vi "PPAS-simulate-dashboard.vi"() -> ()   [LabVIEW 2019]
uses:
  Swerve_Drive_System/PPAS_DRIVE_GLOBALS.vi
  Simulation/PPAS_SIM_SIM_Globals.vi
  AutoCommand/PPAS_AUTOCMD_GLOBALS.vi
  <vilib>/Rock Robotics/WPI/ThirdParty/JAS_Junk/TrajLib/Trajectory_Library.lvlib
  Vision_Interface/PPAS_Vision_Globals.vi
  CommandProcessing/PPAS_Command_Globals.vi
  <vilib>/Rock Robotics/WPI/ThirdParty/JAS_Junk/TrajLib/TypeDef/ROTATION2D.ctl
  <vilib>/Rock Robotics/WPI/ThirdParty/JAS_Junk/TrajLib/TypeDef/CHASSIS_SPEEDS.ctl
  <vilib>/Rock Robotics/WPI/ThirdParty/JAS_Junk/TrajLib/TypeDef/TRANSLATION2D.ctl
  <vilib>/Rock Robotics/WPI/ThirdParty/JAS_Junk/TrajLib/TypeDef/POSE2D.ctl
panel:
  in  "Tab Control":T1(tab)
  out "Mod Swerve in Deadband 2":bool
  out "Battery Voltage":dbl(graph)
  out "Swerve Motor Demands":T2(graph)
  out "Drive Motor Demands":T2(graph)
  out "Swerve Module Devices":T3(array[cluster])
  out "GyroReading_Degreees":dbl format="%15.3f"
  out "Encoder Distances":dbl[](array[numeric]) format="%17.2f"
  out "Encoder Velocities":dbl[](array[numeric]) format="%17.2f"
  out "Motor Demands":dbl[](array[numeric]) format="%17.2f"
  out "Battery Volts":dbl format="%16.2f"
  out "Mod Wheel \nSpeed Dmd":dbl[](array[numeric]) format="%17.3f"
  out "Swerve Drive Motor output":T4(graph)
  out "Swerve Drive Speed M/S":T5(graph)
  out "Swerve Drive Speed Error  M/S":T6(graph)
  out "Closed Loop Control":bool
  out "Orientation Angle Dmd_Rad":dbl format="%17.3f"
  out "Drv Chassis Adj Velocity DmD":T7 {"vOmega" format="%10.3f"; "vY" format="%10.3f"; "vX" format="%10.3f"}
  out "GyroHeading_Radians":dbl format="%17.2f"
  out "Orientation Angle Error_Rad":dbl format="%17.3f"
  out "Orientation Correct CO":dbl format="%17.3f"
  out "Swerve Chassis Speed":T7 {"vOmega" format="%10.3f"; "vY" format="%10.3f"; "vX" format="%10.3f"}
  out "Mod Swerve in Deadband":bool
  out "Mod Wheel Out":dbl[](array[numeric]) format="%17.3f"
  out "Mod Wheel \nSpeed M/S":dbl[](array[numeric]) format="%17.3f"
  out "Mod Wheel Speed Err":dbl[](array[numeric]) format="%17.3f"
  out "Opt Mod Wheel \nSpeed Dmd":dbl[](array[numeric]) format="%17.3f"
  out "Swerve Pos Dmd\nRadians":dbl[](array[numeric]) format="%17.3f"
  out "Optimized Swerve\nPos Dmd":dbl[](array[numeric]) format="%17.3f"
  out "Sweve Module Motor Output":T8(graph)
  out "Swerve Modue Position Radians":T5(graph)
  out "Swerve Module Position Error\nRadians":T9(graph)
  out "Closed Loop Control 2":bool
  out "Mod Swerve in Deadband 3":bool
  out "Mod Swerve Err  Radians":dbl[](array[numeric]) format="%17.3f"
  out "Mod Swerve Motor Out":dbl[](array[numeric]) format="%17.3f"
  out "Mod Pos Radians":dbl[](array[numeric]) format="%17.3f"
  out "Mod Swerve On Targ":bool[](array[boolean])
  out "Cmd 3":bool
  out "Cmd 2":bool
  out "Cmd 1":bool
  out "Vision Pose":T10={"TRANSLATION"={"X"=0.0, "Y"=0.0}, "ROTATION"={"VALUE"=0.0, "COS"=1.0, "SIN"=0.0}} {"ROTATION"."SIN" format="%13.4f"; "ROTATION"."COS" format="%13.4f"; "ROTATION"."VALUE" format="%13.4f"; "TRANSLATION"."Y" format="%14.3f"; "TRANSLATION"."X" format="%14.3f"}
  out "Vision\nPose":bool
  out "Trajectory Status":T13(graph)
  out "Trajectory Execution \nClosed Loop":bool
  out "Mod Swerve in \nDeadband 3":bool
  out "Trajectory Error":T14(graph)
  out "Traj_OnTarget":bool
  out "Traj Heading Dmd Deg":dbl format="%17.2f"
  out "Traj Final Heading Dmd Deg":dbl format="%17.2f"
  out "Traj Sample Time Sec":dbl format="%17.2f"
  out "Traj Rot Vel FF Rad/Sec":dbl format="%17.2f"
  out "Absolute Odometry \nPose":T10={"TRANSLATION"={"X"=0.0, "Y"=0.0}, "ROTATION"={"VALUE"=0.0, "COS"=1.0, "SIN"=0.0}} {"ROTATION"."SIN" format="%13.4f"; "ROTATION"."COS" format="%13.4f"; "ROTATION"."VALUE" format="%13.4f"; "TRANSLATION"."Y" format="%14.3f"; "TRANSLATION"."X" format="%14.3f"}
  out "Other ABS Odometry\nPose":T10={"TRANSLATION"={"X"=0.0, "Y"=0.0}, "ROTATION"={"VALUE"=0.0, "COS"=1.0, "SIN"=0.0}} {"ROTATION"."SIN" format="%13.4f"; "ROTATION"."COS" format="%13.4f"; "ROTATION"."VALUE" format="%13.4f"; "TRANSLATION"."Y" format="%14.3f"; "TRANSLATION"."X" format="%14.3f"}
  # "SIMULATION"
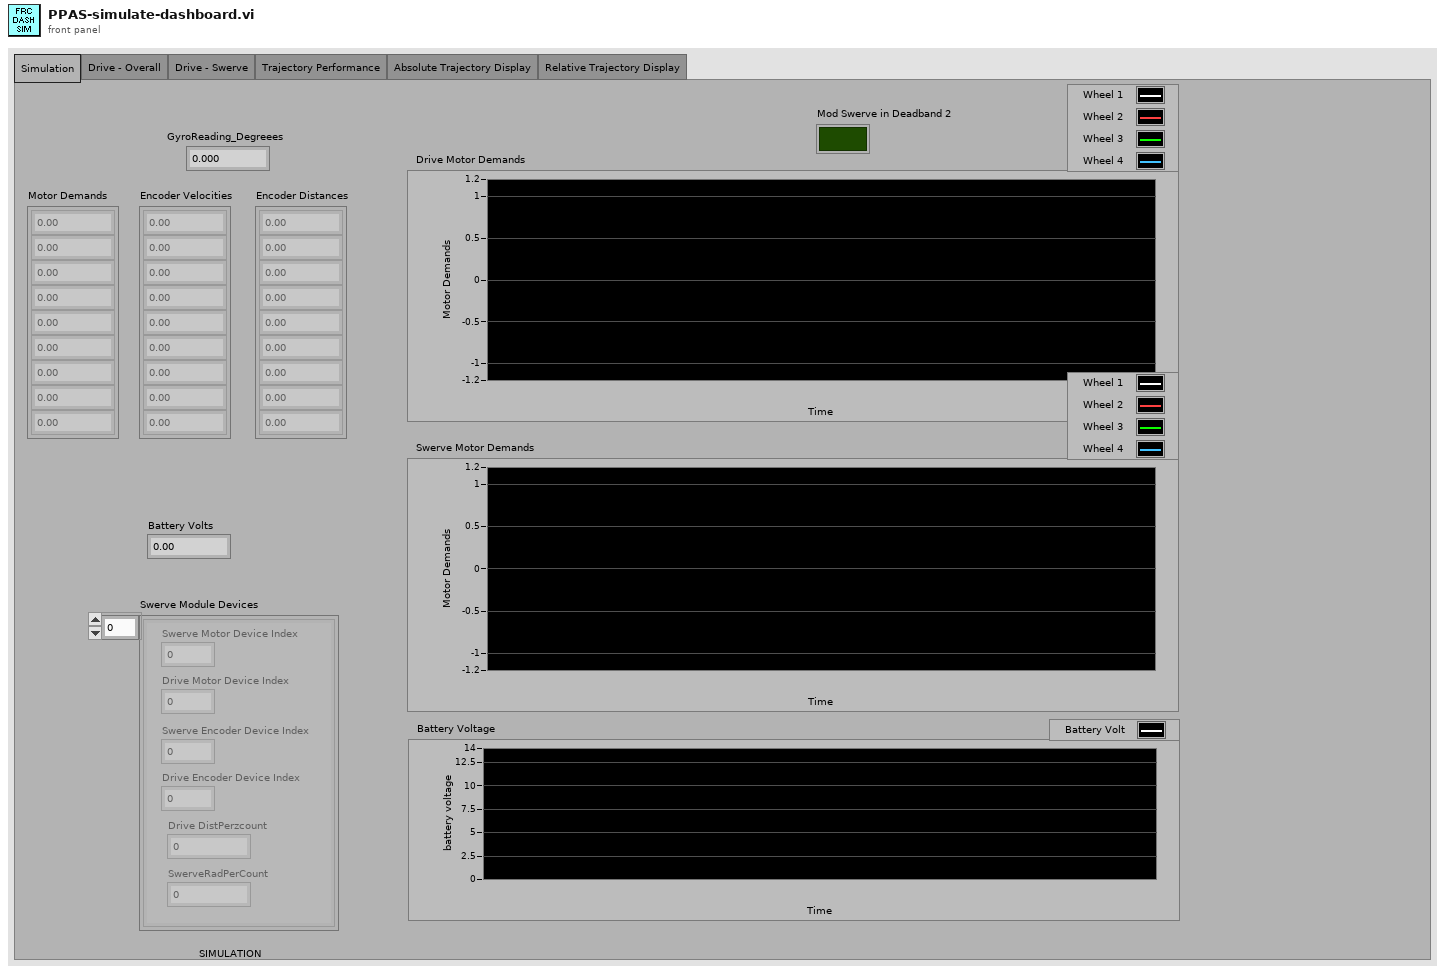
[diagram p1: front panel]
types:
  T1 = enum32{"Simulation", "Drive - Overall", "Drive - Swerve", "Trajectory Performance", "Absolute Trajectory Display", "Relative Trajectory Display"}
  T2 = cluster{"Motor Dmd":dbl, "Motor Dmd":dbl, "Motor Dmd":dbl, "Motor Dmd":dbl}
  T3 = cluster{"Swerve Motor Device Index":i32, "Drive Motor Device Index":i32, "Swerve Encoder Device Index":i32, "Drive Encoder Device Index":i32, "Drive DistPerzcount":dbl, "SwerveRadPerCount":dbl}[]
  T4 = cluster{"Mod Wheel Out[0]":dbl, "Mod Wheel Out[1]":dbl, "Mod Wheel Out[2]":dbl, "Mod Wheel Out[3]":dbl}
  T5 = cluster{"Angle RADIANS":dbl, "Angle RADIANS":dbl, "Angle RADIANS":dbl, "Distance M":dbl}
  T6 = cluster{"Mod Wheel Speed Err[0]":dbl, "Mod Wheel Speed Err[1]":dbl, "Mod Wheel Speed Err[2]":dbl, "Mod Wheel Speed Err[3]":dbl}
  T7 = typedef "Trajectory_Library.lvlib/CHASSIS_SPEEDS.ctl" = cluster{"vX":dbl, "vY":dbl, "vOmega":dbl}
  T8 = cluster{"Mod Swerve Out[0]":dbl, "Mod Swerve Out[1]":dbl, "Mod Swerve Out[2]":dbl, "Mod Swerve Out[3]":dbl}
  T9 = cluster{"Mod Swerve Err[0]":dbl, "Mod Swerve Err[1]":dbl, "Mod Swerve Err[2]":dbl, "Mod Swerve Err[3]":dbl}
  T10 = typedef "Trajectory_Library.lvlib/POSE2D.ctl" = cluster{"TRANSLATION":T11, "ROTATION":T12}
  T11 = typedef "Trajectory_Library.lvlib/TRANSLATION2D.ctl" = cluster{"X":dbl, "Y":dbl}
  T12 = typedef "Trajectory_Library.lvlib/ROTATION2D.ctl" = cluster{"VALUE":dbl, "COS":dbl, "SIN":dbl}
  T13 = cluster{dbl, dbl, dbl, "Traj_Sample_Time_Sec":dbl}
  T14 = cluster{"Traj X Err":dbl, "Traj Y Err":dbl, "Traj Heading Err":dbl}
  T15 = cluster{"Traj X Err_FT":dbl, "Traj Y Err_FT":dbl, "Traj Heading Err_DEG":dbl}
  T16 = typedef "Trajectory_Library.lvlib/SWERVE_DRIVE_MODULE_POSITION.ctl" = cluster{"Distance":dbl, "Angle":T12, "P":bool}
  T17 = typedef "Trajectory_Library.lvlib/SWERVE_DRIVE_MODULE_STATE.ctl" = cluster{"Speed":dbl, "Angle":T12}
  T18 = cluster{"Angle RADIANS":dbl, "Angle RADIANS":dbl, "Angle RADIANS":dbl, "Angle RADIANS":dbl}
  T19 = cluster{"Speed M/S":dbl, "Speed M/S":dbl, "Speed M/S":dbl, "Speed M/S":dbl}
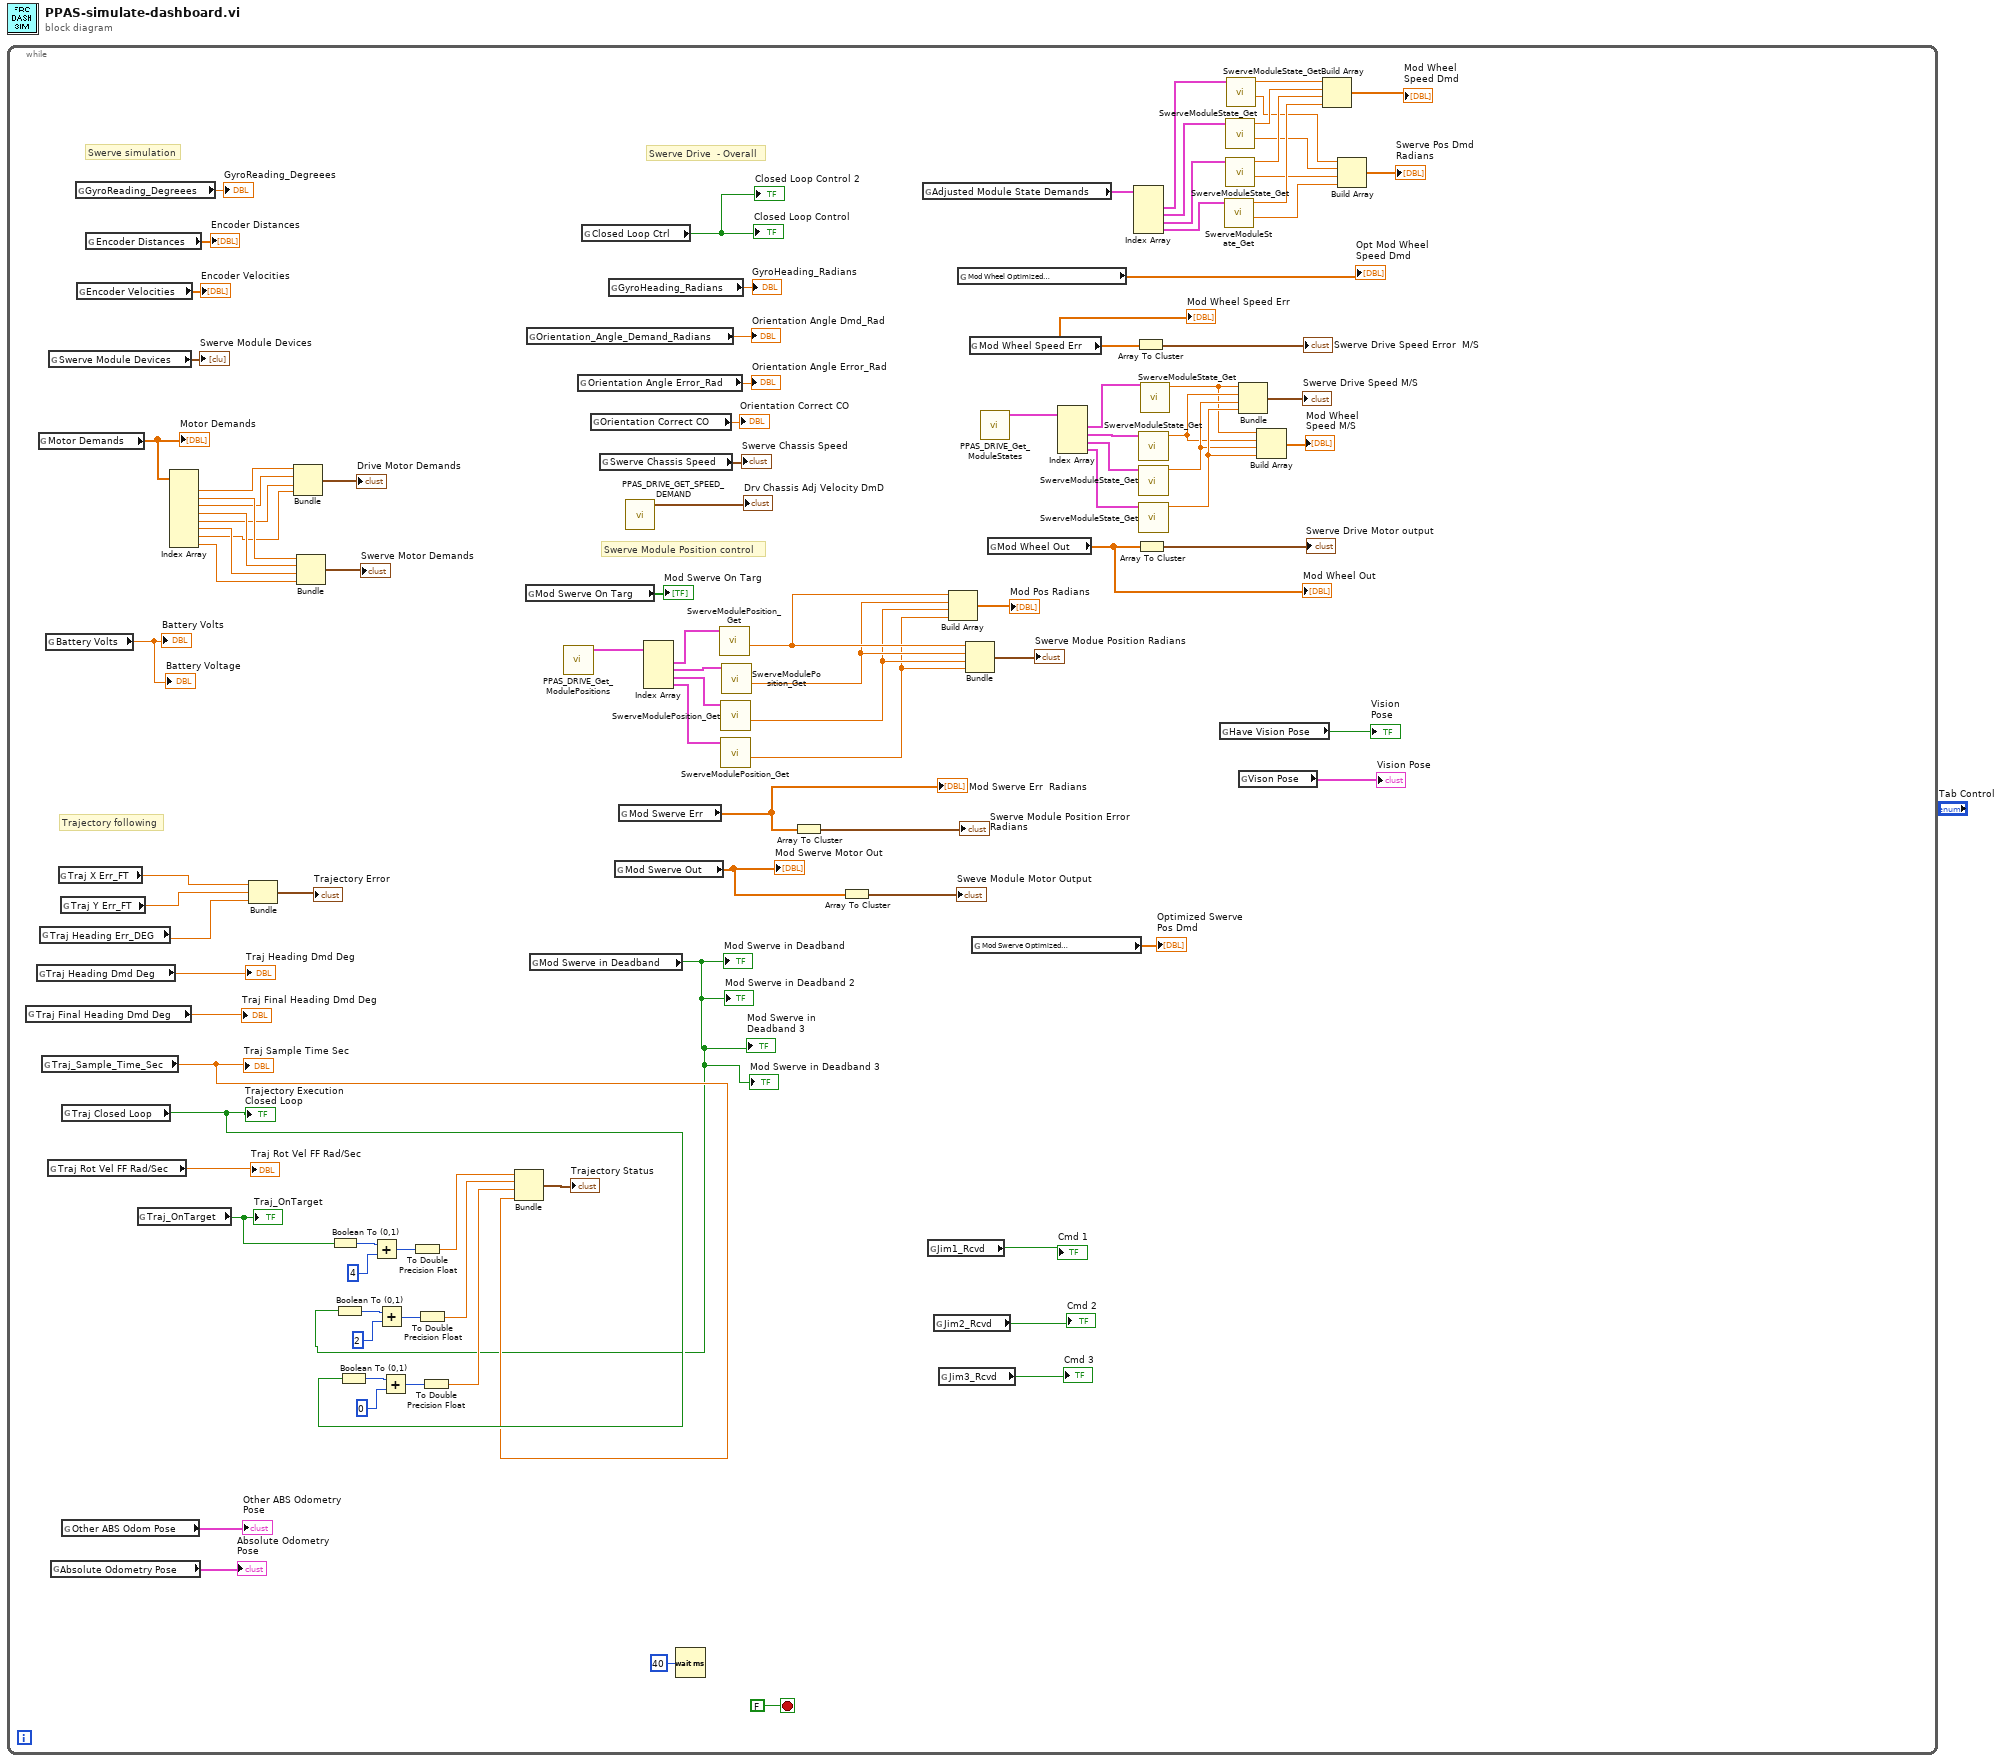
[diagram p0: block diagram]
diagram:
  n1 = while {
    stop <- FALSE stop-if-true
    # "Swerve Module Position control"
    # "Trajectory following"
    # "Swerve simulation"
    # "Swerve Drive  - Overall"
    n2 = global read "PPAS_AUTOCMD_GLOBALS.vi" "Traj Final Heading Dmd Deg"() -> (→"Traj Final Heading Dmd Deg":dbl)
    n3 = global read "PPAS_AUTOCMD_GLOBALS.vi" "Traj Heading Dmd Deg"() -> (→"Traj Heading Dmd Deg":dbl)
    n4 = global read "PPAS_SIM_SIM_Globals.vi" "Motor Demands"() -> (w91:dbl[])
    "Motor Demands" <- w91
    n5 = global read "PPAS_AUTOCMD_GLOBALS.vi" "Traj Heading Err_DEG"() -> (w78:dbl)
    n6 = global read "PPAS_AUTOCMD_GLOBALS.vi" "Traj_Sample_Time_Sec"() -> (w59:dbl)
    "Traj Sample Time Sec" <- w59
    n7 = global read "PPAS_SIM_SIM_Globals.vi" "Battery Volts"() -> (→"Battery Volts" →"Battery Voltage":dbl)
    n8 = global read "PPAS_AUTOCMD_GLOBALS.vi" "Traj Rot Vel FF Rad/Sec"() -> (→"Traj Rot Vel FF Rad/Sec":dbl)
    n9 = global read "PPAS_SIM_SIM_Globals.vi" "Swerve Module Devices"() -> (→"Swerve Module Devices":T3)
    n10 = global read "PPAS_AUTOCMD_GLOBALS.vi" "Absolute Odometry Pose"() -> (→"Absolute Odometry \nPose":T10)
    n11 = global read "PPAS_AUTOCMD_GLOBALS.vi" "Traj X Err_FT"() -> (w80:dbl)
    n12 = global read "PPAS_AUTOCMD_GLOBALS.vi" "Traj Y Err_FT"() -> (w79:dbl)
    n13 = global read "PPAS_AUTOCMD_GLOBALS.vi" "Traj Closed Loop"() -> (w61:bool)
    "Trajectory Execution \nClosed Loop" <- w61
    n14 = global read "PPAS_AUTOCMD_GLOBALS.vi" "Other ABS Odom Pose"() -> (→"Other ABS Odometry\nPose":T10)
    n15 = global read "PPAS_SIM_SIM_Globals.vi" "GyroReading_Degreees"() -> (→"GyroReading_Degreees":dbl)
    n16 = global read "PPAS_SIM_SIM_Globals.vi" "Encoder Velocities"() -> (→"Encoder Velocities":dbl[])
    n17 = global read "PPAS_SIM_SIM_Globals.vi" "Encoder Distances"() -> (→"Encoder Distances":dbl[])
    n18 = global read "PPAS_AUTOCMD_GLOBALS.vi" "Traj_OnTarget"() -> (w73:bool)
    "Traj_OnTarget" <- w73
    n19 = Index Array(array=w91) -> (element #1=w90:dbl, element #2=w89:dbl, element #3=w88:dbl, element #4=w87:dbl, element #5=w86:dbl, element #6=w85:dbl, element #7=w84:dbl, element #8=w83:dbl)  [unwired: 8 in]
    n20 = Bundle("Traj X Err_FT"=w80, "Traj Y Err_FT"=w79, "Traj Heading Err_DEG"=w78) -> (→"Trajectory Error":T15)  [unwired: 1 in]
    n21 = Bundle("Motor Dmd"=w90, "Motor Dmd"=w88, "Motor Dmd"=w86, "Motor Dmd"=w84) -> (→"Drive Motor Demands":T2)  [unwired: 1 in]
    n22 = Bundle("Motor Dmd"=w89, "Motor Dmd"=w87, "Motor Dmd"=w85, "Motor Dmd"=w83) -> (→"Swerve Motor Demands":T2)  [unwired: 1 in]
    n23 = Boolean To (0,1)(Boolean=w73) -> (0, 1=w71:i16)
    n24 = Boolean To (0,1)(Boolean=w61) -> (0, 1=w64:i16)
    n25 = Add(x=w71, y=i16 4) -> (x+y=w70:i16)
    n26 = Add(x=w64, y=i16 0) -> (x+y=w63:i16)
    n27 = To Double Precision Float(number=w70) -> (double precision float=w72:dbl)
    n28 = To Double Precision Float(number=w63) -> (double precision float=w60:dbl)
    n29 = global read "PPAS_DRIVE_GLOBALS.vi" "Mod Swerve On Targ"() -> (→"Mod Swerve On Targ":bool[])
    n30 = global read "PPAS_DRIVE_GLOBALS.vi" "Orientation_Angle_Demand_Radians"() -> (→"Orientation Angle Dmd_Rad":dbl)
    n31 = global read "PPAS_DRIVE_GLOBALS.vi" "Mod Swerve in Deadband"() -> (w46:bool)
    "Mod Swerve in Deadband" <- w46
    "Mod Swerve in Deadband 2" <- w46
    "Mod Swerve in \nDeadband 3" <- w46
    "Mod Swerve in Deadband 3" <- w46
    n32 = Boolean To (0,1)(Boolean=w46) -> (0, 1=w68:i16)
    n33 = Add(x=w68, y=i16 2) -> (x+y=w67:i16)
    n34 = To Double Precision Float(number=w67) -> (double precision float=w65:dbl)
    n35 = Bundle(w72, w65, w60, "Traj_Sample_Time_Sec"=w59) -> (→"Trajectory Status":T13)  [unwired: 1 in]
    n36 = call "PPAS_DRIVE_Get_ModulePositions.vi"() -> ("Swerve Module Positions"=w55:T16[])  [unwired: 11 in]
    n37 = global read "PPAS_DRIVE_GLOBALS.vi" "Orientation Angle Error_Rad"() -> (→"Orientation Angle Error_Rad":dbl)
    n38 = global read "PPAS_DRIVE_GLOBALS.vi" "Closed Loop Ctrl"() -> (→"Closed Loop Control" →"Closed Loop Control 2":bool)
    n39 = global read "PPAS_DRIVE_GLOBALS.vi" "Orientation Correct CO"() -> (→"Orientation Correct CO":dbl)
    n40 = global read "PPAS_DRIVE_GLOBALS.vi" "Swerve Chassis Speed"() -> (→"Swerve Chassis Speed":T7)
    n41 = global read "PPAS_DRIVE_GLOBALS.vi" "GyroHeading_Radians"() -> (→"GyroHeading_Radians":dbl)
    n42 = global read "PPAS_DRIVE_GLOBALS.vi" "Mod Swerve Out"() -> (w34:dbl[])
    "Mod Swerve Motor Out" <- w34
    n43 = global read "PPAS_DRIVE_GLOBALS.vi" "Mod Swerve Err"() -> (w50:dbl[])
    "Mod Swerve Err  Radians" <- w50
    n44 = call "PPAS_DRIVE_GET_SPEED_DEMAND.vi"() -> ("Drv Chassis Velocity DmD"=→"Drv Chassis Adj Velocity DmD":T7)  [unwired: 11 in]
    n45 = Index Array(array=w55) -> (element #1=w54:T16, element #2=w53:T16, element #3=w52:T16, element #4=w51:T16)  [unwired: 4 in]
    n46 = Wait (ms)(milliseconds to wait=u32 40) -> ()  [unwired: 1 out]
    n47 = call <vilib>:"SwerveModulePosition_Get.vi"("Swerve Module Position"=w54) -> ("Angle RADIANS"=w33:dbl)  [unwired: 8 in, 2 out]
    n48 = call <vilib>:"SwerveModulePosition_Get.vi"("Swerve Module Position"=w52) -> ("Angle RADIANS"=w31:dbl)  [unwired: 8 in, 2 out]
    n49 = call <vilib>:"SwerveModulePosition_Get.vi"("Swerve Module Position"=w51) -> ("Angle RADIANS"=w30:dbl)  [unwired: 8 in, 2 out]
    n50 = call <vilib>:"SwerveModulePosition_Get.vi"("Swerve Module Position"=w53) -> ("Angle RADIANS"=w32:dbl)  [unwired: 8 in, 2 out]
    n51 = Array To Cluster(array=w50) -> (cluster=→"Swerve Module Position Error\nRadians":T9)
    n52 = Array To Cluster(array=w34) -> (cluster=→"Sweve Module Motor Output":T8)
    n53 = global read "PPAS_DRIVE_GLOBALS.vi" "Adjusted Module State Demands"() -> (w23:T17[])
    n54 = global read "PPAS_Command_Globals.vi" "Jim1_Rcvd"() -> (→"Cmd 1":bool)
    n55 = global read "PPAS_Command_Globals.vi" "Jim2_Rcvd"() -> (→"Cmd 2":bool)
    n56 = global read "PPAS_Command_Globals.vi" "Jim3_Rcvd"() -> (→"Cmd 3":bool)
    n57 = Build Array(w33, w32, w31, w30) -> (→"Mod Pos Radians":dbl[])
    n58 = global read "PPAS_DRIVE_GLOBALS.vi" "Mod Wheel Optimized \nDmd"() -> (→"Opt Mod Wheel \nSpeed Dmd":dbl[])
    n59 = Bundle("Angle RADIANS"=w33, "Angle RADIANS"=w32, "Angle RADIANS"=w31, "Angle RADIANS"=w30) -> (→"Swerve Modue Position Radians":T18)  [unwired: 1 in]
    n60 = global read "PPAS_DRIVE_GLOBALS.vi" "Mod Wheel Speed Err"() -> (w49:dbl[])
    "Mod Wheel Speed Err" <- w49
    n61 = global read "PPAS_DRIVE_GLOBALS.vi" "Mod Swerve Optimized\nDmd"() -> (→"Optimized Swerve\nPos Dmd":dbl[])
    n62 = call "PPAS_DRIVE_Get_ModuleStates.vi"() -> ("Swerve Module States"=w43:T17[])  [unwired: 11 in]
    n63 = global read "PPAS_DRIVE_GLOBALS.vi" "Mod Wheel Out"() -> (w37:dbl[])
    "Mod Wheel Out" <- w37
    n64 = Index Array(array=w43) -> (element #1=w41:T17, element #2=w42:T17, element #3=w40:T17, element #4=w39:T17)  [unwired: 4 in]
    n65 = Index Array(array=w23) -> (element #1=w22:T17, element #2=w21:T17, element #3=w20:T17, element #4=w19:T17)  [unwired: 4 in]
    n66 = Array To Cluster(array=w49) -> (cluster=→"Swerve Drive Speed Error  M/S":T6)
    n67 = Array To Cluster(array=w37) -> (cluster=→"Swerve Drive Motor output":T4)
    n68 = call <vilib>:"SwerveModuleState_Get.vi"("Desired State"=w42) -> ("Speed M/S"=w25:dbl)  [unwired: 9 in, 1 out]
    n69 = call <vilib>:"SwerveModuleState_Get.vi"("Desired State"=w40) -> ("Speed M/S"=w26:dbl)  [unwired: 9 in, 1 out]
    n70 = call <vilib>:"SwerveModuleState_Get.vi"("Desired State"=w39) -> ("Speed M/S"=w27:dbl)  [unwired: 9 in, 1 out]
    n71 = call <vilib>:"SwerveModuleState_Get.vi"("Desired State"=w41) -> ("Speed M/S"=w24:dbl)  [unwired: 9 in, 1 out]
    n72 = global read "PPAS_Vision_Globals.vi" "Have Vision Pose"() -> (→"Vision\nPose":bool)
    n73 = call <vilib>:"SwerveModuleState_Get.vi"("Desired State"=w19) -> ("Angle RADIANS"=w9:dbl, "Speed M/S"=w15:dbl)  [unwired: 9 in]
    n74 = call <vilib>:"SwerveModuleState_Get.vi"("Desired State"=w21) -> ("Angle RADIANS"=w11:dbl, "Speed M/S"=w17:dbl)  [unwired: 9 in]
    n75 = call <vilib>:"SwerveModuleState_Get.vi"("Desired State"=w20) -> ("Angle RADIANS"=w10:dbl, "Speed M/S"=w16:dbl)  [unwired: 9 in]
    n76 = call <vilib>:"SwerveModuleState_Get.vi"("Desired State"=w22) -> ("Angle RADIANS"=w12:dbl, "Speed M/S"=w18:dbl)  [unwired: 9 in]
    n77 = Bundle("Speed M/S"=w24, "Speed M/S"=w25, "Speed M/S"=w26, "Speed M/S"=w27) -> (→"Swerve Drive Speed M/S":T19)  [unwired: 1 in]
    n78 = global read "PPAS_Vision_Globals.vi" "Vison Pose"() -> (→"Vision Pose":T10)
    n79 = Build Array(w24, w25, w26, w27) -> (→"Mod Wheel \nSpeed M/S":dbl[])
    n80 = Build Array(w18, w17, w16, w15) -> (→"Mod Wheel \nSpeed Dmd":dbl[])
    n81 = Build Array(w12, w11, w10, w9) -> (→"Swerve Pos Dmd\nRadians":dbl[])
  }
